vi "Connect.vi"(8 "error in (no error)":errorcluster, 10 "Connection String":string, 11 "SQLConnection Type":refnum<class "DBC.lvclass">) -> (0 "error out":errorcluster, 3 "SQLConnection out":refnum<class "DBC.lvclass">)   [LabVIEW 2020, in "ORM_DBC_Mssql.lvlib" / "DBC.lvclass"]
uses:
  DBC.lvclass
  C:/Program Files/National Instruments/LabVIEW 2024/vi.lib/Viviota/shared/ORM_DBC_dotNet.lvlibp/dbcDotNet/ORM_DBC_dotNet.lvclass
  C:/Program Files/National Instruments/LabVIEW 2024/vi.lib/Viviota/shared/ORM.lvlibp/ORM/DbConnection/DbConnection.lvclass
  System.Data
  <vilib>/Viviota/shared/ORM_DBC_dotNet.lvlibp/dbcDotNet/Write connection.vi
  <vilib>/Viviota/shared/ORM.lvlibp/ORM/DbConnection/Write ColumnNameEqualsValueFormat.vi
  <vilib>/Viviota/shared/ORM.lvlibp/ORM/DbConnection/Write ColumnNameFormat.vi
  <vilib>/Viviota/shared/ORM.lvlibp/ORM/DbConnection/Write LastIdentityQuery.vi
  <vilib>/Viviota/shared/ORM.lvlibp/ORM/DbConnection/Write SupportBulkCreate.vi
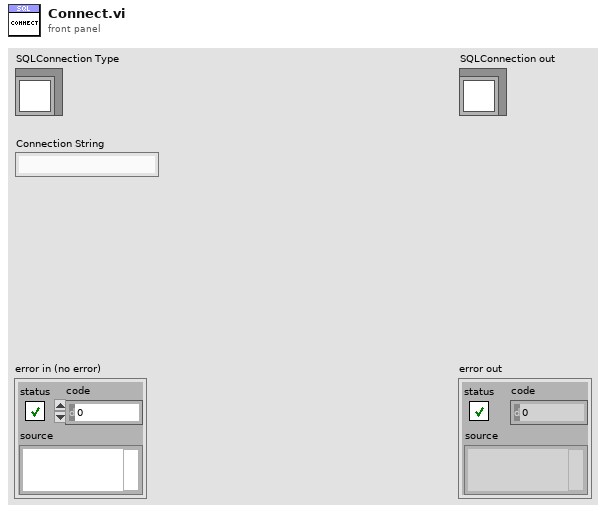
[diagram p1: front panel]
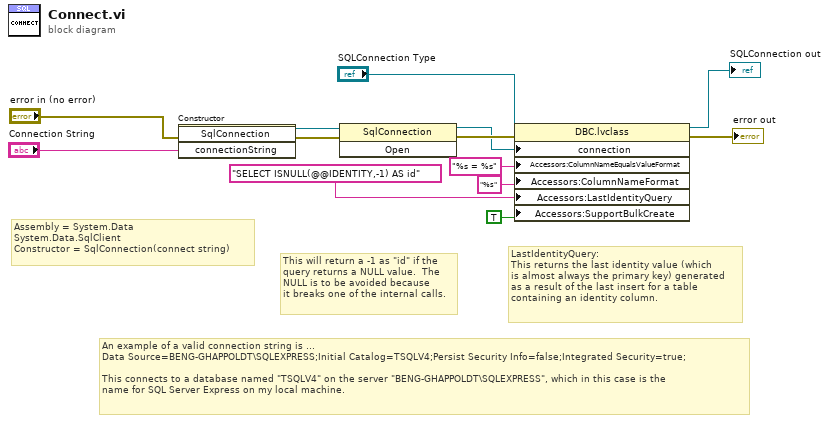
[diagram p0: block diagram]
diagram:
  # "An example of a valid connection string is ...\nData Source=BENG-GHAPPOLDT\\SQLEXPRESS;Initial Catalog=TSQLV4;Persist Security Info=false;Integrated Security=true; \n\nThis connects to a database named \"TSQLV4\" on the server \"BENG-GHAPPOLDT\\SQLEXPRESS\", which in this case is the\nname for SQL Server Express on my local machine."
  # "LastIdentityQuery:\nThis returns the last identity value (which\nis almost always the primary key) generated\nas a result of the last insert for a table \ncontaining an identity column."
  # "Assembly = System.Data\nSystem.Data.SqlClient\nConstructor = SqlConnection(connect string)"
  # "This will return a -1 as \"id\" if the\nquery returns a NULL value.  The\nNULL is to be avoided because\nit breaks one of the internal calls."
  n1 = constructor class="SqlConnection"(error in="error in (no error)", "connectionString"="Connection String") -> (reference out=w11:refnum<k24>, error out=w10:errorcluster)  [unwired: 2 in, 2 out]
  n2 = invoke class="SqlConnection" method="Open"(reference=w11, error in=w10) -> (reference out=w7:refnum<k24>, error out=w8:errorcluster)  [unwired: 1 in, 1 out]
  n3 = property class="DBC.lvclass"(reference="SQLConnection Type", error in=w8, "connection"=w7, "Accessors:ColumnNameEqualsValueFormat"="%s = %s" ("ColumnNameEqualsValueFormat"), "Accessors:ColumnNameFormat"="%s" ("ColumnNameFormat"), "Accessors:LastIdentityQuery"="SELECT ISNULL(@@IDENTITY,-1) AS id" ("LastIdentityQuery"), "Accessors:SupportBulkCreate"=TRUE ("SupportBulkCreate")) -> (reference out=→"SQLConnection out":refnum<class "DBC.lvclass">, error out=→"error out":errorcluster)
